vi "client.vi"() -> ()   [LabVIEW 2019]
uses:
  Generated_client/RPC Messages/Greeter_MessageA.ctl
  Generated_client/RPC Messages/Greeter_req.ctl
  Generated_client/RPC Messages/Greeter_req_req_oneof/Greeter_req_req_oneof.lvclass
  Generated_client/RPC Messages/Greeter_req_req_oneof/Greeter_req_req_oneof.lvclass/Greeter_req_req_oneof.ctl
  Generated_client/RPC Messages/Greeter_res_res_oneof/Greeter_res_res_oneof.lvclass/Greeter_res_res_oneof.ctl
  Generated_client/Generated_client.lvlib
  Generated_client/RPC Messages/Greeter_res_res_oneof/Greeter_res_res_oneof.lvclass
panel:
  out "name_res":string
  out "data_resp":T1
  out "res_id":i32
  in  "Use MessageA?":bool
  in  "data_a1":string="abc"
  in  "req_name":string="Dann"
  in  "req_id":dbl=101.0
  out "error out":errorcluster
  in  "error in":errorcluster
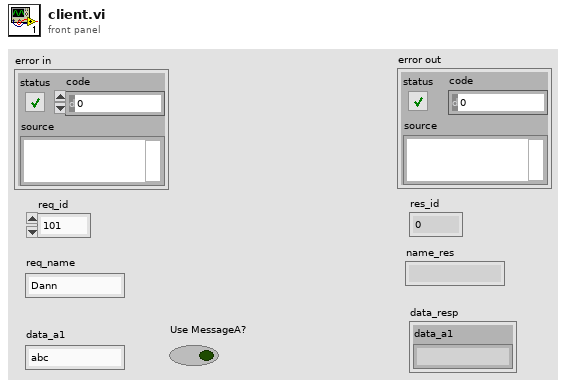
[diagram p1: front panel]
types:
  T1 = typedef "Generated_client.lvlib/Greeter_MessageA.ctl" = cluster{"data_a1":string}
  T2 = typedef "Generated_client.lvlib/Greeter_req.ctl" = cluster{"req_id":i32, "Greeter_req_req_oneof":refnum<class "Greeter_req_req_oneof.lvclass">}
  T3 = typedef "grpc-lvsupport-release.lvlib/grpcId.ctl" = u64
  T4 = typedef "Generated_client.lvlib/Greeter_res.ctl" = cluster{"res_id":i32, "Greeter_res_res_oneof":refnum<class "Greeter_res_res_oneof.lvclass">}
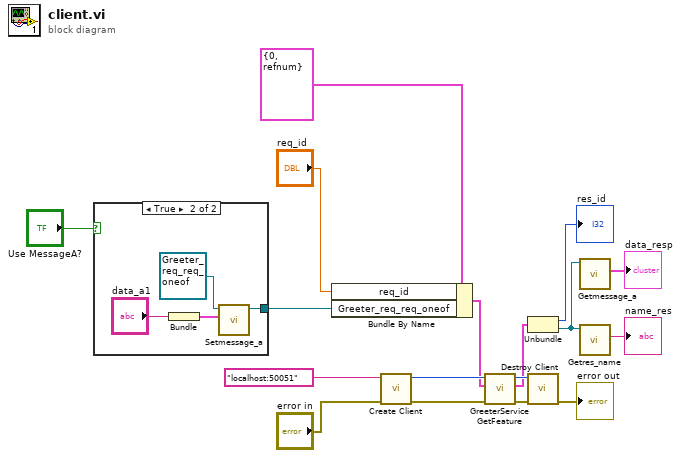
[diagram p0: block diagram]
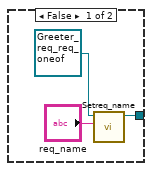
[diagram p2: hidden frame]
diagram:
  n1 = case shown="True" "Use MessageA?" {
    tunnel: [w19 w21] -> w8
    frame False {
      n2 = call "Setreq_name.vi"("Set_Val"="req_name", "OneOfTemplate in"=refnum<class "Greeter_req_req_oneof.lvclass"> refnum) -> ("OneOfTemplate out"=w19:refnum<class "Greeter_req_req_oneof.lvclass">)  [unwired: 8 in, 1 out]
    }
    frame True {
      n3 = Bundle("data_a1"="data_a1") -> (w23:cluster{"data_a1":string})  [unwired: 1 in]
      n4 = call "Setmessage_a.vi"("Set_Val"=w23, "OneOfTemplate in"=refnum<class "Greeter_req_req_oneof.lvclass"> refnum) -> ("OneOfTemplate out"=w21:refnum<class "Greeter_req_req_oneof.lvclass">)  [unwired: 8 in, 1 out]
    }
  }
  n5 = Bundle By Name(cluster=T2 {"req_id"=0, "Greeter_req_req_oneof"=refnum} ("Greeter_req"), "req_id"="req_id", "Greeter_req_req_oneof"=w8) -> (w6:T2)
  n6 = call "Create Client.vi"("error in"="error in", "address"="localhost:50051") -> ("error out"=w16:errorcluster, "gRPC ID Out"=w13:T3)  [unwired: 8 in]
  n7 = call "GreeterService GetFeature.vi"("error in"=w16, "Request Data"=w6, "gRPC ID"=w13) -> ("error out"=w15:errorcluster, "Response Data"=w5:T4, "gRPC ID out"=w14:T3)  [unwired: 6 in]
  n8 = Unbundle(w5) -> ("res_id"=→"res_id":i32, "Greeter_res_res_oneof"=w3:refnum<class "Greeter_res_res_oneof.lvclass">)
  n9 = call "Destroy Client.vi"("error in"=w15, "gRPC ID"=w14) -> ("error out"=→"error out":errorcluster)  [unwired: 9 in]
  n10 = call "Getmessage_a.vi"("OneOfTemplate in"=w3) -> ("Get_Val"=→"data_resp":T1)  [unwired: 8 in, 2 out]
  n11 = call "Getres_name.vi"("OneOfTemplate in"=w3) -> ("Get_Val"=→"name_res":string)  [unwired: 8 in, 2 out]
